vi "GenerateCommand.vi"(10 "DataIn":u8[](array[numeric]) format="%x") -> (2 "Command":string)   [LabVIEW 2013]
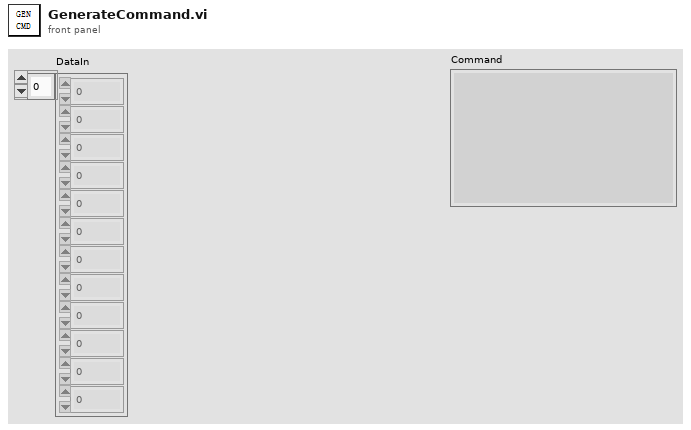
[diagram p1: front panel]
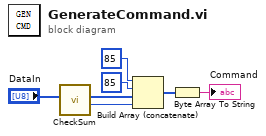
[diagram p0: block diagram]
diagram:
  n1 = call "CheckSum.vi"("DataIn"="DataIn") -> ("CheckSum"=w3:u8, "DataOut"=w4:u8[])  [unwired: 9 in]
  n2 = Build Array (concatenate)(u8 85, u8 85, w4, w3) -> (w1:u8[])
  n3 = Byte Array To String(unsigned byte array=w1) -> (string=→"Command":string)
